vi "DC Voltmeter.vi"() -> ()   [LabVIEW 2009]
uses:
  <vilib>/DAQmx/read.llb/DAQmx Read (Analog 1D DBL 1Chan NSamp).vi
  <vilib>/DAQmx/configure/timing.llb/DAQmx Timing (Sample Clock).vi
  <vilib>/DAQmx/create/channels.llb/DAQmx Create Channel (AI-Voltage-Basic).vi
  <vilib>/Utility/file.llb/Write To Spreadsheet File (DBL).vi
  <vilib>/Analysis/NI_AALBase.lvlib
panel:
  out "ScanGraph":cluster{dbl[], dbl[]}(graph)
  in  "Save?":bool
  in  "Scan Save Path":path
  in  "?":bool
  out "Mean Voltage Channel A":dbl format="%#.4f"
  in  "Input Voltage A":tag
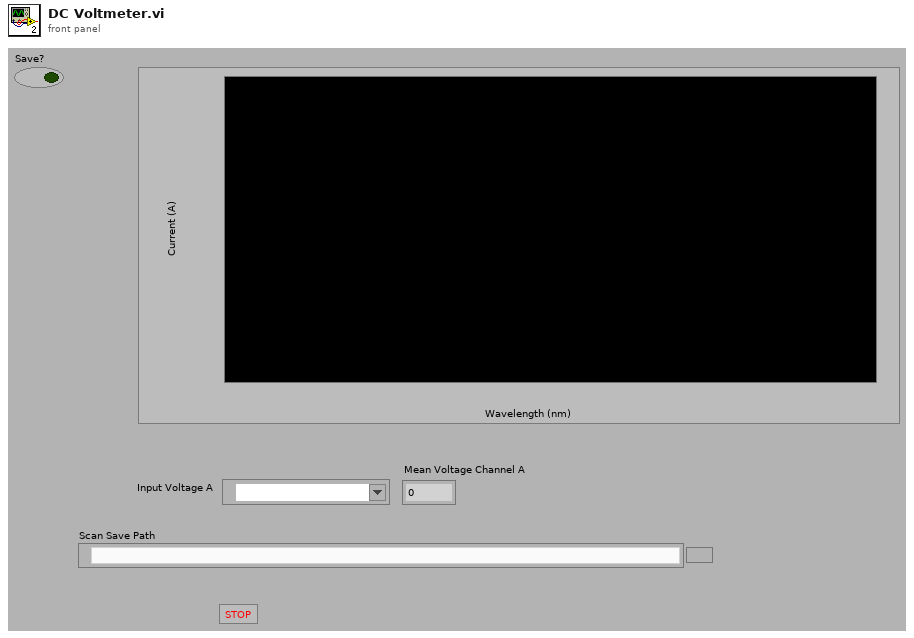
[diagram p1: front panel]
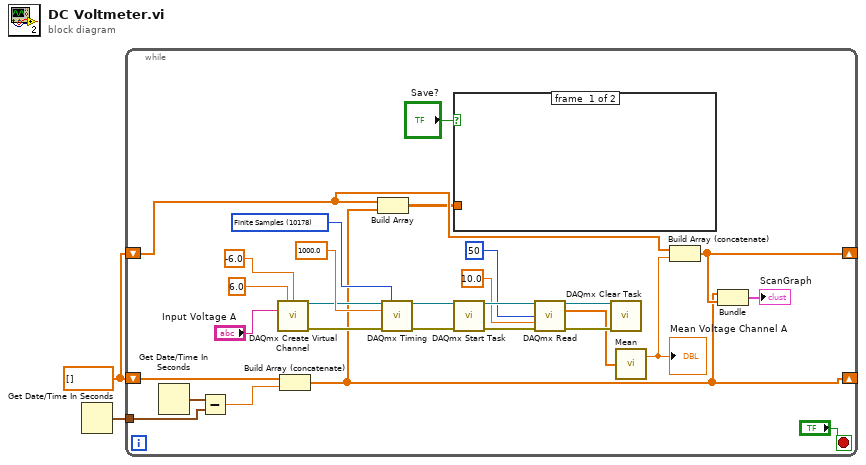
[diagram p0: block diagram]
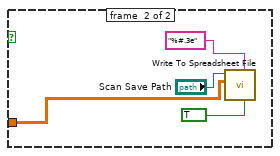
[diagram p2: hidden frame]
diagram:
  w1 = dbl[] [] ("data")
  n1 = Get Date/Time In Seconds() -> (seconds since 1Jan1904=w2:timestamp)
  n2 = while {
    shift-right: [w7] -> _
    shift-left: w1 -> [w5]
    tunnel: w2 -> [w11]
    shift-right: [w4] -> _
    shift-left: w1 -> [w9]
    stop <- "?" stop-if-true
    w27 = 10178 items=["Finite Samples"=10178, "Continuous Samples"=10123, "Hardware Timed Single Point"=12522] ("sample mode")
    n3 = Get Date/Time In Seconds() -> (seconds since 1Jan1904=w12:timestamp)
    n4 = Subtract(x=w12, y=w11) -> (x-y=w8:dbl)
    n5 = call-poly <vilib>:"DAQmx Create Virtual Channel.vi"("maximum value"=6.0, "minimum value"=-6.0 ("maximum value"), "physical channels"="Input Voltage A") -> ("task out"=w16:refnum<k21>, "error out"=w15:errorcluster)  [unwired: 6 in, 5 out]
    n6 = Build Array (concatenate)(w9, w8) -> (w4:dbl[])
    n7 = Build Array(w5, w4) -> (w3:dbl[][])
    n8 = call-poly <vilib>:"DAQmx Timing.vi"("task/channels in"=w16, "sample mode"=w27, "rate"=1000.0, "error in"=w15) -> ("task out"=w26:refnum<k21>, "error out"=w25:errorcluster)  [unwired: 3 in, 7 out]
    n9 = case shown="True" "Save?" {
      tunnel: w3 -> [_ w31]
      frame #0 {
      }
      frame #1 {
        n10 = call-poly <vilib>:"Write To Spreadsheet File.vi"("transpose? (no:F)"=TRUE, "format (%.3f)"="%#.3e", "2D data"=w31, "file path (dialog if empty)"="Scan Save Path") -> ()  [unwired: 4 in, 1 out]
      }
    }
    n11 = call <vilib>:"DAQmx Start Task.vi"("task/channels in"=w26, "error in"=w25) -> ("task out"=w24:refnum<k21>, "error out"=w23:errorcluster)  [unwired: 12 out]
    n12 = call-poly <vilib>:"DAQmx Read.vi"("task/channels in"=w24, "number of samples per channel"=50, "timeout"=10.0, "error in"=w23) -> ("task out"=w21:refnum<k21>, "data"=w13:dbl[], "error out"=w20:errorcluster)  [unwired: 9 out]
    n13 = call <vilib>:"DAQmx Clear Task.vi"("task in"=w21, "error in"=w20) -> ()  [unwired: 14 out]
    n14 = call <vilib>:"Mean.vi"("X"=w13) -> ("mean"=w10:dbl)  [unwired: 1 out]
    "Mean Voltage Channel A" <- w10
    n15 = Build Array (concatenate)(w5, w10) -> (w7:dbl[])
    n16 = Bundle(w4, w7) -> (→"ScanGraph":cluster{dbl[], dbl[]})  [unwired: 1 in]
  }
